vi "Create LabView Wizard Dir.vi"   [LabVIEW 2012, in "Application.lvlib"]
uses:
  Application.lvlib
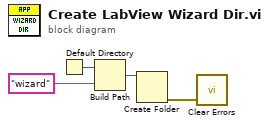
[diagram p0: block diagram]
diagram:
  n1 = Default Directory() -> (w4:path)
  n2 = Build Path(base path=w4, name or relative path="wizard" ("名称或相对路径")) -> (appended path=w2:path)
  n3 = Create Folder(path (use dialog)=w2) -> (error out=w1:errorcluster)  [unwired: 2 in, 2 out]
  n4 = call <vilib>:"Clear Errors.vi"("error in (no error)"=w1) -> ()  [unwired: 6 in, 1 out]
